vi "moving average.vi"(1 "length":i32=10, 2 "raw array":dbl[](array[numeric])) -> (0 "averaged array":dbl[](array[numeric]))   [LabVIEW 2017]
uses:
  <vilib>/Analysis/baseanly.llb/Mean (DBL).vi
  <vilib>/Analysis/NI_AALBase.lvlib
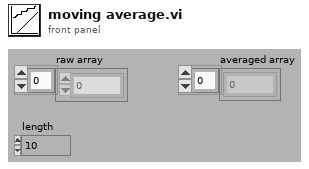
[diagram p1: front panel]
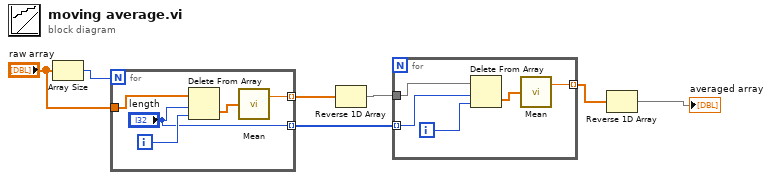
[diagram p0: block diagram]
diagram:
  n1 = Array Size(array="raw array") -> (size(s)=w6:i32)
  n2 = for {
    N: w6 -> [_]
    tunnel: "raw array" -> [w12]
    tunnel: [w11] -> w5 mode=indexing
    tunnel: ["length"] -> w3 mode=indexing
    i -> [w9]
    n3 = Delete From Array "Delete From Array"(array=w12, length="length", index=w9) -> (deleted portion=w10:dbl[])  [unwired: 1 out]
    n4 = call-poly <vilib>:"Mean.vi"("X"=w10) -> ("mean"=w11:dbl)  [unwired: 1 out]
  }
  n5 = Reverse 1D Array(array=w5) -> (reversed array=w4:dbl[])
  n6 = for {
    tunnel: w4 -> [w17]
    tunnel: [w16] -> w2 mode=indexing
    tunnel: w3 -> [w13] mode=indexing
    i -> [w14]
    n7 = Delete From Array "Delete From Array"(array=w17, length=w13, index=w14) -> (deleted portion=w15:dbl[])  [unwired: 1 out]
    n8 = call-poly <vilib>:"Mean.vi"("X"=w15) -> ("mean"=w16:dbl)  [unwired: 1 out]
  }
  n9 = Reverse 1D Array(array=w2) -> (reversed array=→"averaged array":dbl[])
